vi "WM_CAP - From fourcc.vi"(7 "FOURCC":string) -> (8 "biCompression":i32 format="%.0x")   [LabVIEW 2022 SP3]
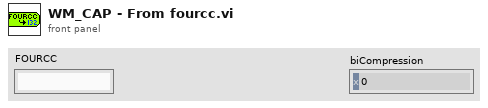
[diagram p1: front panel]
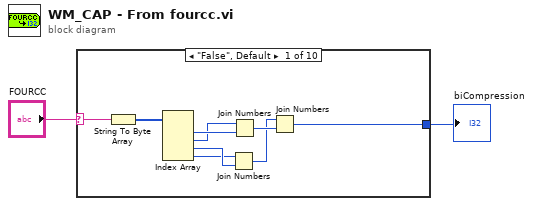
[diagram p0: block diagram]
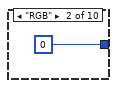
[diagram p2: hidden frame]
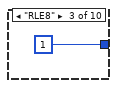
[diagram p3: hidden frame]
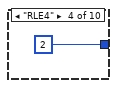
[diagram p4: hidden frame]
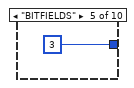
[diagram p5: hidden frame]
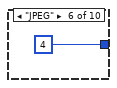
[diagram p6: hidden frame]
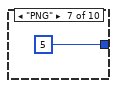
[diagram p7: hidden frame]
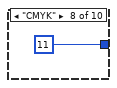
[diagram p8: hidden frame]
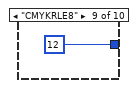
[diagram p9: hidden frame]
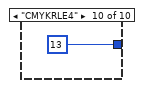
[diagram p10: hidden frame]
diagram:
  n1 = case shown="\"False\", Default" "FOURCC" {
    selector: "FOURCC" -> [w11 _ _ _ _ _ _ _ _ _]
    tunnel: [w9 0 1 2 3 4 5 11 12 13] -> w1
    frame "False", Default {
      n2 = String To Byte Array(string=w11) -> (unsigned byte array=w10:u8[])
      n3 = Index Array(array=w10) -> (element #1=w8:u8, element #2=w7:u8, element #3=w4:u8, element #4=w3:u8)  [unwired: 4 in]
      n4 = Join Numbers(hi=w3, lo=w4) -> ((hi.lo)=w5:u16)
      n5 = Join Numbers(hi=w7, lo=w8) -> ((hi.lo)=w6:u16)
      n6 = Join Numbers(hi=w5, lo=w6) -> ((hi.lo)=w9:u32)
    }
    frame "RGB" {
    }
    frame "RLE8" {
    }
    frame "RLE4" {
    }
    frame "BITFIELDS" {
    }
    frame "JPEG" {
    }
    frame "PNG" {
    }
    frame "CMYK" {
    }
    frame "CMYKRLE8" {
    }
    frame "CMYKRLE4" {
    }
  }
  "biCompression" <- w1
